vi "GetTopicNode_etc.vi"(2 "node":string, 3 "topic":string) -> (1 "Baxter":T2)   [LabVIEW 2010]
uses:
  <userlib>/ROSforLV_0.1/ROS/Code/SubVIs/_ROSControl.ctl
  <userlib>/ROSforLV_0.1/ROS/Code/SubVIs/_ROSDirection.ctl
  <userlib>/ROSforLV_0.1/ROS/Code/_ROSDefinition.vi
panel:
  out "Action":T1
  out "Found?":bool
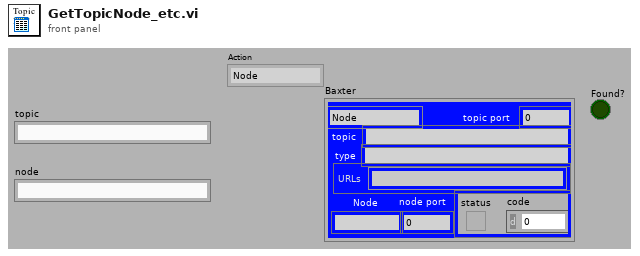
[diagram p1: front panel]
types:
  T1 = typedef "_ROSDirection.ctl" = enum16{"Node", "Publisher", "Subscriber", "Service Client"}
  T2 = typedef "_ROSControl.ctl" = cluster{"topic port":u16, "Node":string, "topic":string, "type":string, "node port":u32, "error ":errorcluster, "Direction":T1, "APIs":string[]}
  T3 = cluster{"Topic":string, "Type":string, "Action":T1}[]
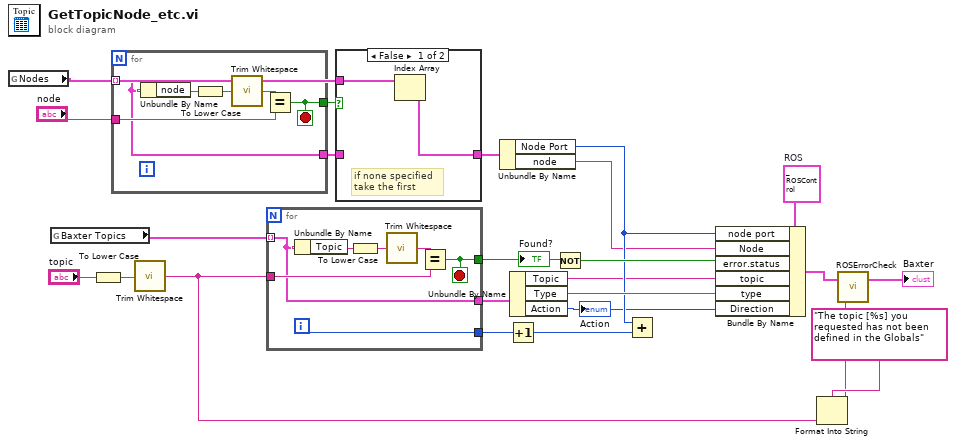
[diagram p0: block diagram]
diagram:
  w5 = T2 {"topic port"=0, "Node"="", "topic"="", "type"="", "node port"=0, "error "={"status"=FALSE, "code"=0, "source"=""}, "Direction"=enum."Node", "APIs"=[]}  # ROS
  n1 = global read "_ROSDefinition.vi" "Nodes"() -> (w3:cluster{"node":string, "Node Port":u32}[])
  n2 = global read "_ROSDefinition.vi" "Baxter Topics"() -> (w4:T3)
  n3 = To Lower Case(string="topic") -> (all lower case string=w24:string)
  n4 = for {
    tunnel: "node" -> [w28]
    tunnel: [w27] -> w17
    tunnel: [w25] -> w15
    tunnel: w3 -> [w25] mode=indexing
    stop <- w27 stop-if-true
    n5 = Unbundle By Name(w25) -> ("node"=w26:string)
    n6 = To Lower Case(string=w26) -> (all lower case string=w30:string)
    n7 = call <vilib>:"Trim Whitespace.vi"("string"=w30) -> ("trimmed string"=w29:string)  [unwired: 1 in]
    n8 = Equal?(x=w29, y=w28) -> (x = y?=w27:bool)
  }
  n9 = call <vilib>:"Trim Whitespace.vi"("string"=w24) -> ("trimmed string"=w6:string)  [unwired: 1 in]
  n10 = for {
    tunnel: w6 -> [w35]
    tunnel: [w34] -> w1
    tunnel: [w32] -> w23
    tunnel: w4 -> [w32] mode=indexing
    tunnel: [w31] -> w13
    i -> [w31]
    stop <- w34 stop-if-true
    n11 = Unbundle By Name(w32) -> ("Topic"=w33:string)
    n12 = To Lower Case(string=w33) -> (all lower case string=w37:string)
    n13 = call <vilib>:"Trim Whitespace.vi"("string"=w37) -> ("trimmed string"=w36:string)  [unwired: 1 in]
    n14 = Equal?(x=w36, y=w35) -> (x = y?=w34:bool)
  }
  "Found?" <- w1
  n15 = case shown="False" w17 {
    tunnel: [w38 w40] -> w16
    tunnel: w15 -> [_ w40]
    tunnel: w3 -> [w39 _]
    frame False {
      # "if none specified\ntake the first"
      n16 = Index Array(array=w39) -> (element=w38:cluster{"node":string, "Node Port":u32})  [unwired: 1 in]
    }
    frame True {
    }
  }
  n17 = Unbundle By Name(w16) -> ("Node Port"=w14:u32, "node"=w11:string)
  n18 = Increment(x=w13) -> (x+1=w12:i32)
  n19 = Unbundle By Name(w23) -> ("Topic"=w8:string, "Type"=w21:string, "Action"=w2:T1)
  "Action" <- w2
  n20 = Not(x=w1) -> (.not. x?=w19:bool)
  n21 = Add(x=w14, y=w12) -> ()  [unwired: 1 out]
  n22 = Bundle By Name(cluster=w5, "node port"=w14, "Node"=w11, "error.status"=w19, "topic"=w8, "type"=w21, "Direction"=w2) -> (w10:T2)
  n23 = Format Into String(format string="The topic [%s] you requested has not been defined in the Globals" ("message"), w6) -> (resulting string=w7:string)  [unwired: 2 in, 1 out]
  n24 = call <userlib>:"ROSErrorCheck.vi"("message"=w7, "ROS in"=w10) -> ("ROS out"=→"Baxter":T2)  [unwired: 1 in]
